vi "TIRF Find EPI.vi"(8 "error in (no error)":errorcluster, 11 "Config In":T1 {"Hardware Configuration"."Lasers Configuration"."SettingValues"."785 Power" format="%.1f"; "Hardware Configuration"."Lasers Configuration"."SettingValues"."647 Power" format="%.1f"; "Hardware Configuration"."Lasers Configuration"."SettingValues"."561 Power" format="%.1f"}) -> (0 "error out":errorcluster, 3 "Config Out":T1 {"Hardware Configuration"."Lasers Configuration"."SettingValues"."785 Power" format="%.1f"; "Hardware Configuration"."Lasers Configuration"."SettingValues"."647 Power" format="%.1f"; "Hardware Configuration"."Lasers Configuration"."SettingValues"."561 Power" format="%.1f"})   [LabVIEW 2020]
uses:
  Settings/System Running Settings.ctl
  Support/Hardware Configuration.ctl
  Support/Camera Configuration.ctl
  controls/ROI.ctl
  D:/Daguan/Development/RM21-MMicrosopeSource/HardwareAdapter/Camera/Dependencies/PVCamNET.dll
  Camera/Dependencies/PVCamNET.dll
  <vilib>/vision/Image Controls.llb/IMAQ Image.ctl
  D:/Daguan/Development/RM21-MMicrosopeSource/HardwareAdapter/Lasers/Dependencies/Oxxius_Boxx.dll
  Lasers/Dependencies/Oxxius_Boxx.dll
  Logging/Logging Configuration.ctl
  controls/DeviceStatusCtl.ctl
  controls/CallBack Refs.ctl
  Dependencies/MicroDrive.dll
  Logging/Logging.lvlib
  Settings/Settings.lvlib
panel:
  out "Current Position":dbl
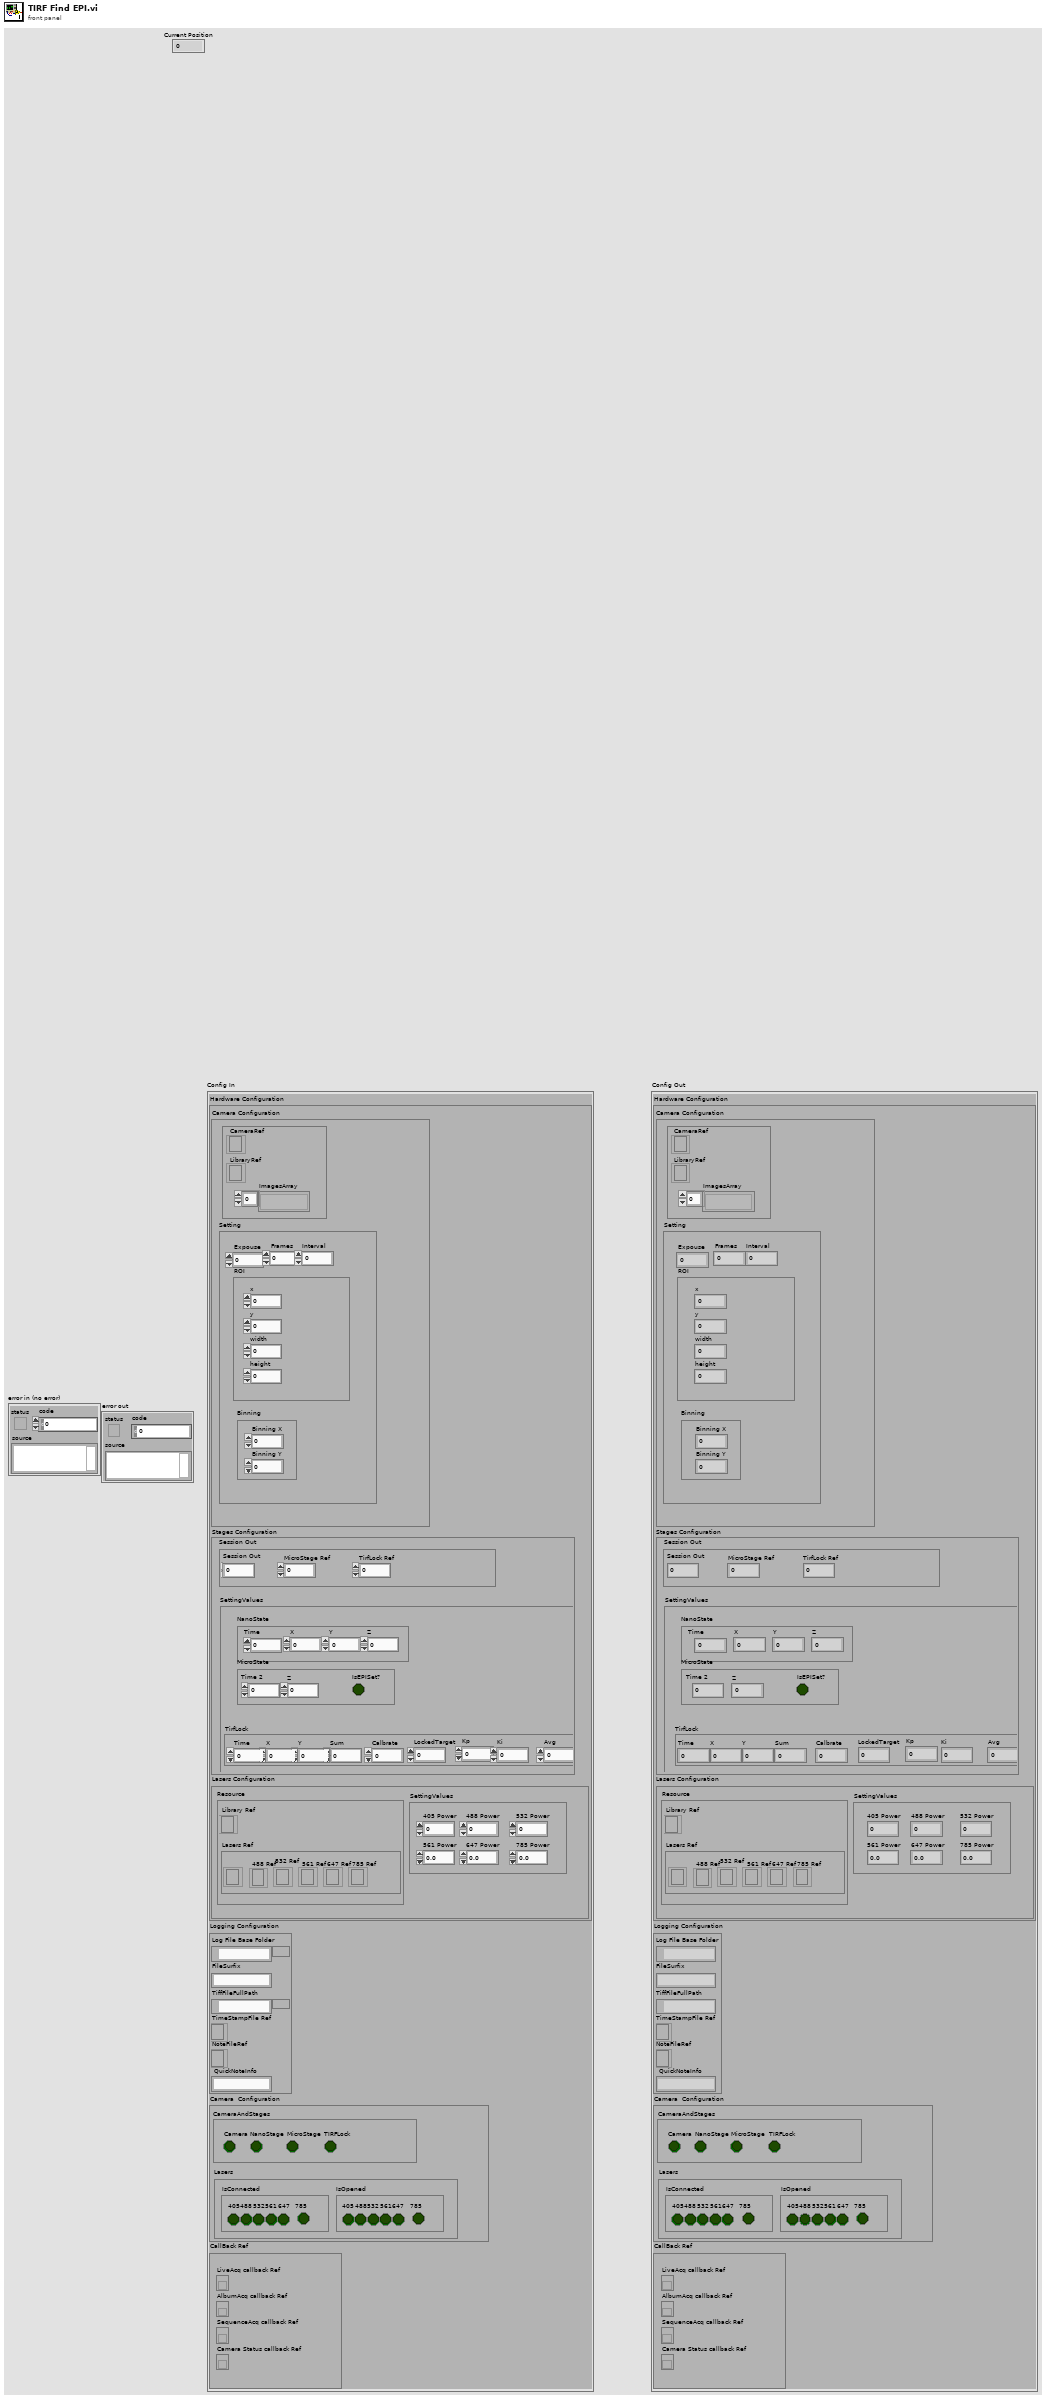
[diagram p1: front panel]
types:
  T1 = typedef "Settings.lvlib/System Running Settings.ctl" = cluster{"Hardware Configuration":T2, "Logging Configuration":T6, "HardWare Status":cluster{"CameraAndStages":T7, "Lasers":cluster{"IsConnected":cluster{"405":bool, "488":bool, "532":bool, "561":bool, "647":bool, "785":bool}, "IsOpened":cluster{"405":bool, "488":bool, "532":bool, "561":bool, "647":bool, "785":bool}}}, "CallBack Ref":T8}
  T2 = typedef "Hardware Configuration.ctl" = cluster{"Camera Configuration":T3, "Stages Configuration":cluster{"Resource":cluster{"NanoStage Ref":i32, "MicroStage Ref":i32, "TirfLock Ref":i32}, "SettingValues":cluster{"NanoState":cluster{"Time":dbl, "X":dbl, "Y":dbl, "Z":dbl}, "MicroState":cluster{"Time 2":dbl, "Z":dbl, "IsEPISet?":bool}, "TirfLock":cluster{"Time":dbl, "X":dbl, "Y":dbl, "Sum":dbl, "Calbrate":dbl, "LockedTarget":dbl, "Kp":dbl, "Ki":dbl, "Avg":dbl}}}, "Lasers Configuration":cluster{"SettingValues":cluster{"405 Power":sgl, "488 Power":sgl, "532 Power":sgl, "561 Power":sgl, "647 Power":sgl, "785 Power":sgl}, "Resource":cluster{"Library Ref":refnum<k24>, "Lasers Ref":cluster{"405 Ref":refnum<k24>, "488 Ref":refnum<k24>, "532 Ref":refnum<k24>, "561 Ref":refnum<k24>, "647 Ref":refnum<k24>, "785 Ref":refnum<k24>}}}}
  T3 = typedef "Camera Configuration.ctl" = cluster{"Setting":cluster{"Expouse":dbl, "Frames":dbl, "Interval":dbl, "ROI":T4, "Binning":cluster{"Binning X":dbl, "Binning Y":dbl}}, "Resource":cluster{"CameraRef":refnum<k24>, "LibraryRef":refnum<k24>, "ImagesArray":T5[]}}
  T4 = typedef "ROI.ctl" = cluster{"x":dbl, "y":dbl, "width":dbl, "height":dbl}
  T5 = typedef "IMAQ Image.ctl" = refnum<image>
  T6 = typedef "Logging.lvlib/Logging Configuration.ctl" = cluster{"Log File Base Folder":path, "FileSurfix":string, "TiffFileFullPath":path, "TimeStampFile Ref":refnum<file>, "NoteFileRef":refnum<file>, "QuickNoteInfo":string}
  T7 = typedef "DeviceStatusCtl.ctl" = cluster{"Camera":bool, "NanoStage":bool, "MicroStage":bool, "TIRFLock":bool}
  T8 = typedef "CallBack Refs.ctl" = cluster{"LiveAcq callback Ref":refnum<k27>, "AlbumAcq callback Ref":refnum<k27>, "SequenceAcq callback Ref":refnum<k27>, "Camera Status callback Ref":refnum<k27>}
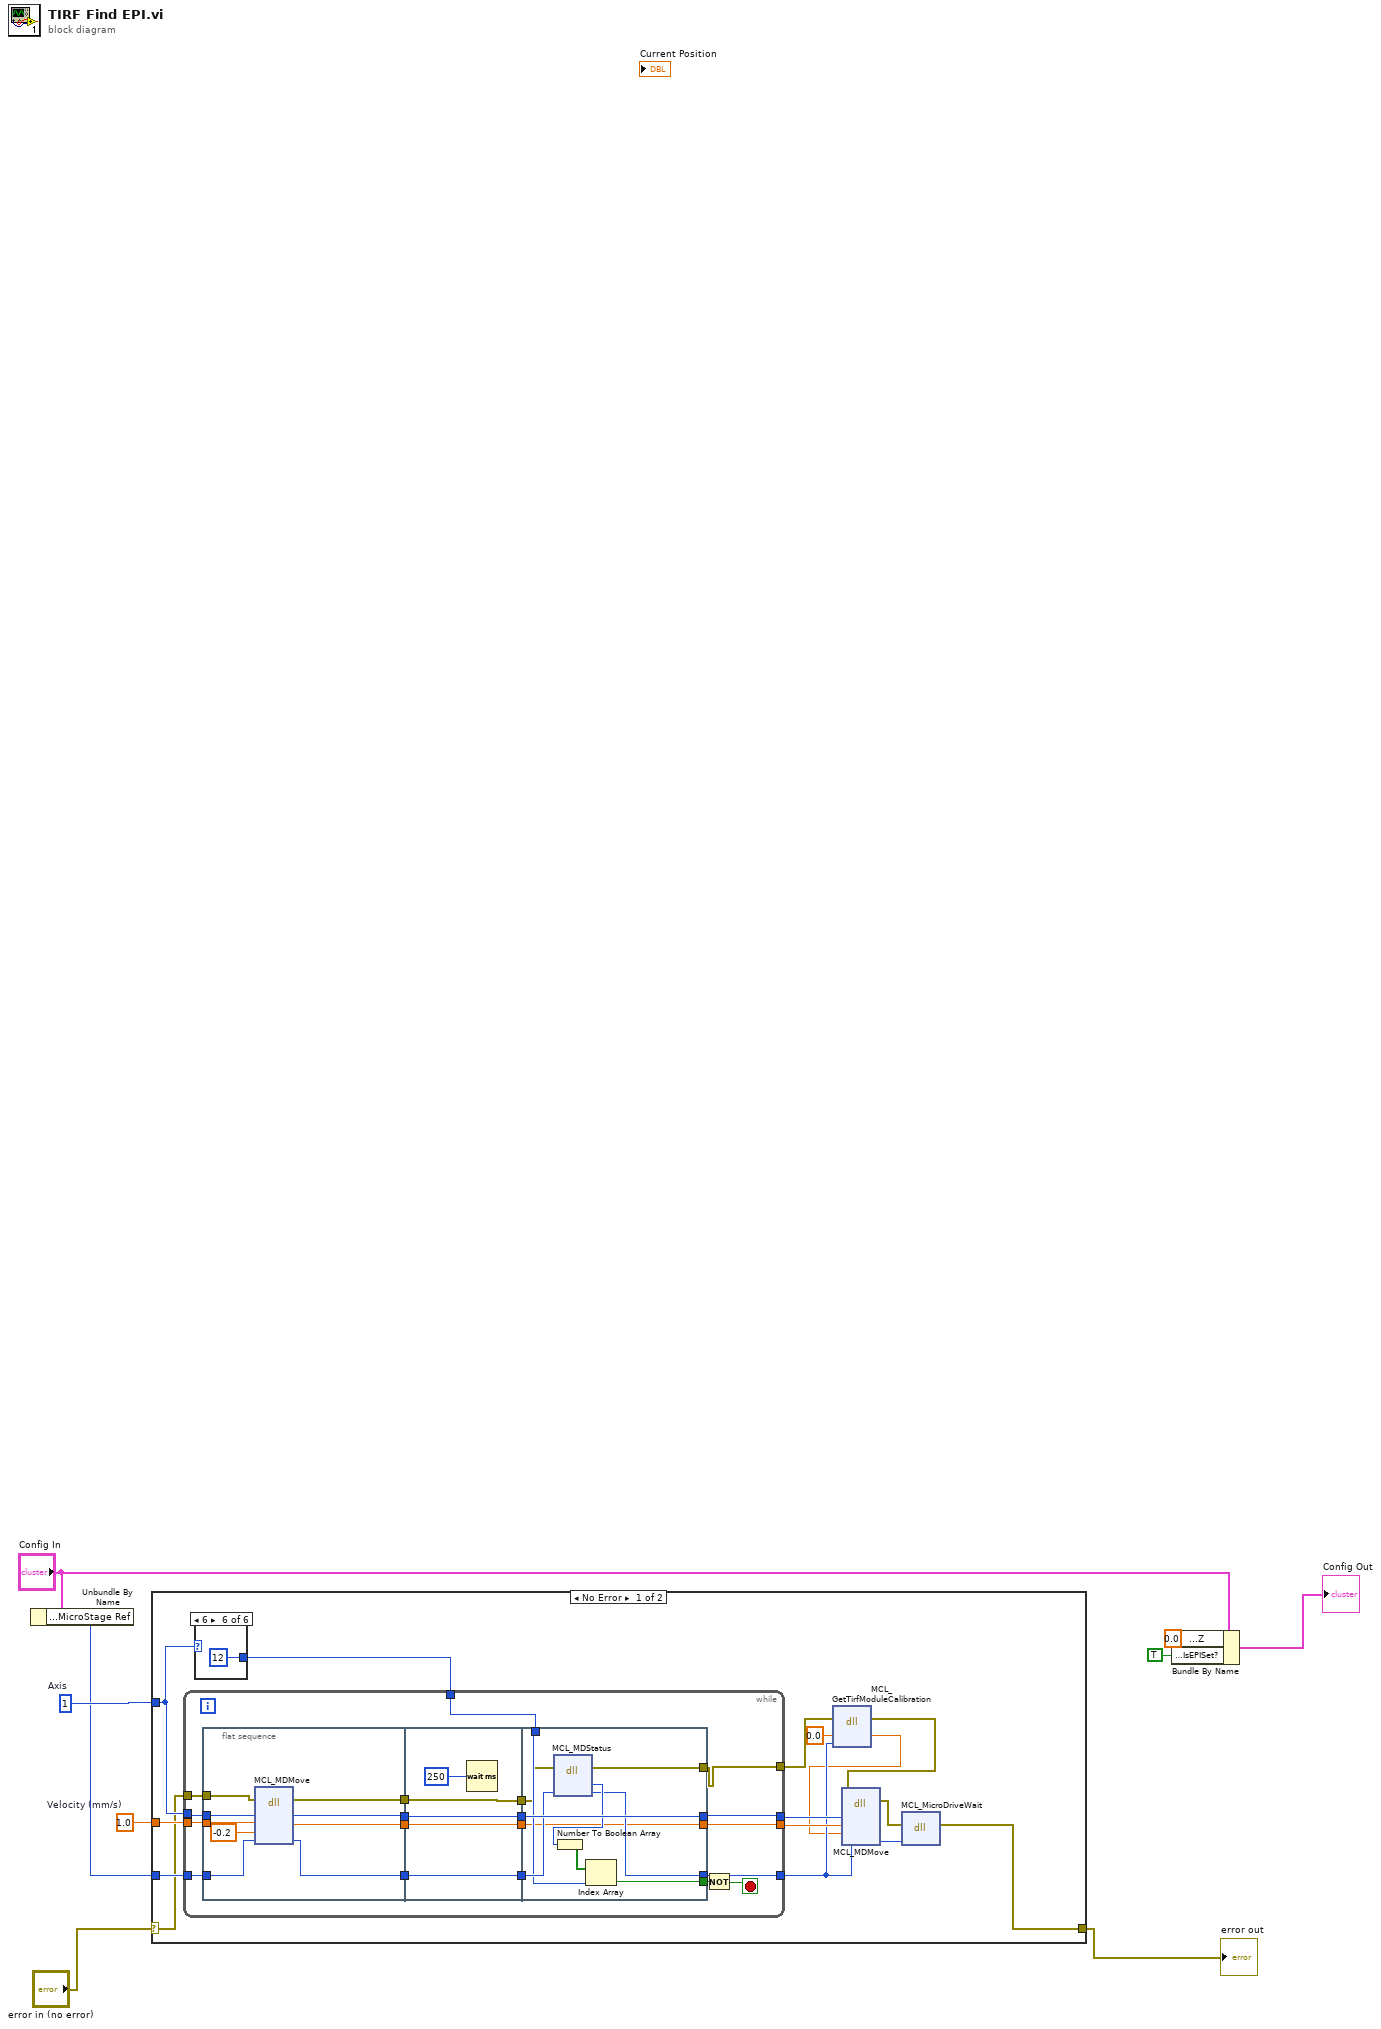
[diagram p0: block diagram]
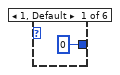
[diagram p2: hidden frame]
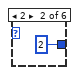
[diagram p3: hidden frame]
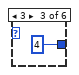
[diagram p4: hidden frame]
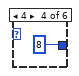
[diagram p5: hidden frame]
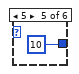
[diagram p6: hidden frame]
diagram:
  w9 = 1.0  # Velocity (mm/s)
  w6 = u16 1  # Axis
  n1 = Unbundle By Name("Config In") -> ("Hardware Configuration.Stages Configuration.Resource.MicroStage Ref"=w5:i32)
  n2 = case shown="No Error" "error in (no error)" {
    selector: "error in (no error)" -> [w14 w74]
    tunnel: w9 -> [w24 _]
    tunnel: w5 -> [w23 _]
    tunnel: w6 -> [w20 _]
    tunnel: [w10 w74] -> w7
    frame No Error {
      n3 = case shown="6" w20 {
        tunnel: [0 2 4 8 10 12] -> w19
        frame 1, Default {
        }
        frame 2 {
        }
        frame 3 {
        }
        frame 4 {
        }
        frame 5 {
        }
        frame 6 {
        }
      }
      n4 = while {
        tunnel: w24 -> [w49]
        tunnel: w23 -> [w45]
        tunnel: [w44] -> w16
        tunnel: w20 -> [w47]
        tunnel: [w46] -> w22
        tunnel: w19 -> [w39]
        tunnel: [w35] -> w18
        tunnel: w14 -> [w34]
        tunnel: [w31] -> w13
        stop <- w48 stop-if-true
        n5 = flat-sequence {
          tunnel: w49 -> [w58]
          tunnel: w47 -> [w56]
          tunnel: w45 -> [w54]
          tunnel: [w55] -> w43
          tunnel: [w53] -> w42
          tunnel: [w52] -> w37
          tunnel: w34 -> [w51]
          tunnel: [w50] -> w33
          tunnel: w43 -> [w63]
          tunnel: w42 -> [w62]
          tunnel: [w63] -> w41
          tunnel: [w62] -> w40
          tunnel: w37 -> [w60]
          tunnel: [w60] -> w36
          tunnel: w33 -> [w59]
          tunnel: [w59] -> w32
          tunnel: [w69] -> w44
          tunnel: [w73] -> w46
          tunnel: w41 -> [w73]
          tunnel: w40 -> [w70]
          tunnel: w39 -> [w68]
          tunnel: [w67] -> w38
          tunnel: w36 -> [w66]
          tunnel: [w66] -> w35
          tunnel: w32 -> [w65]
          tunnel: [w64] -> w31
          frame #0 {
            n6 = dll-call lib="D:/Daguan/Development/RM21-MMicrosopeSource/HardwareAdapter/Stages/Dependencies/MicroDrive.dll" fn="MCL_MDMove"(error in=w51, "axis"=w56, "velocity"=w58, "distance"=-0.2, "handle"=w54) -> (error out=w50:errorcluster, "axis"=w55:i32, "velocity"=w52:dbl, "handle"=w53:i32)  [unwired: 3 in, 2 out]
          }
          frame #1 {
            n7 = Wait (ms)(milliseconds to wait=u32 250) -> ()  [unwired: 1 out]
          }
          frame #2 {
            n8 = dll-call lib="D:/Daguan/Development/RM21-MMicrosopeSource/HardwareAdapter/Stages/Dependencies/MicroDrive.dll" fn="MCL_MDStatus"(error in=w65, "handle"=w70) -> (error out=w64:errorcluster, "status"=w72:u16, "handle"=w69:i32)  [unwired: 2 in, 3 out]
            n9 = Number To Boolean Array(number=w72) -> (Boolean array=w71:bool[])
            n10 = Index Array(array=w71, index=w68) -> (element=w67:bool)
          }
        }
        n11 = Not(x=w38) -> (.not. x?=w48:bool)
      }
      n12 = dll-call lib="D:/Daguan/Development/RM21-MMicrosopeSource/HardwareAdapter/Stages/Dependencies/MicroDrive.dll" fn="MCL_GetTirfModuleCalibration"(error in=w13, "calMM"=0.0 ("distance"), "handle"=w16) -> (error out=w12:errorcluster, "calMM"=w15:dbl)  [unwired: 3 in, 2 out]
      n13 = dll-call lib="D:/Daguan/Development/RM21-MMicrosopeSource/HardwareAdapter/Stages/Dependencies/MicroDrive.dll" fn="MCL_MDMove"(error in=w12, "axis"=w22, "velocity"=w18, "distance"=w15, "handle"=w16) -> (error out=w11:errorcluster, "handle"=w21:i32)  [unwired: 4 in, 3 out]
      n14 = dll-call lib="D:/Daguan/Development/RM21-MMicrosopeSource/HardwareAdapter/Stages/Dependencies/MicroDrive.dll" fn="MCL_MicroDriveWait"(error in=w11, "handle"=w21) -> (error out=w10:errorcluster)  [unwired: 3 in, 2 out]
    }
    frame Error {
    }
  }
  "error out" <- w7
  n15 = Bundle By Name(cluster="Config In", "Hardware Configuration.Stages Configuration.SettingValues.MicroState.Z"=0.0, "Hardware Configuration.Stages Configuration.SettingValues.MicroState.IsEPISet?"=TRUE) -> (→"Config Out":T1)
